vi "GUI_Frog_HPD_imagetester.vi"() -> ()   [LabVIEW 2013]
uses:
  Shared/GUI_Template/GUI_master/tcp_new_data_event.ctl
  Shared/GUI_Template/GUI_master/tcp new data cluster.ctl
  <vilib>/vision/Image Controls.llb/IMAQ Image.ctl
panel:
  out "www":T1(plugin-control)
  in  "retrievedFrogTrace::1":string caption="frogTrace::1"
  in  "frogTrace::1":string
  in  "triggermode::1":bool caption="Blank Button"
  out "test":T1(plugin-control) caption="Retrieved Frog Trace"
  in  "insert tag":bool=TRUE
  in  "stop":bool
  in  "GUIdevice 1":string="FrogHPD"
  out "tcp data event":T2
  out "error IO 2":errorcluster
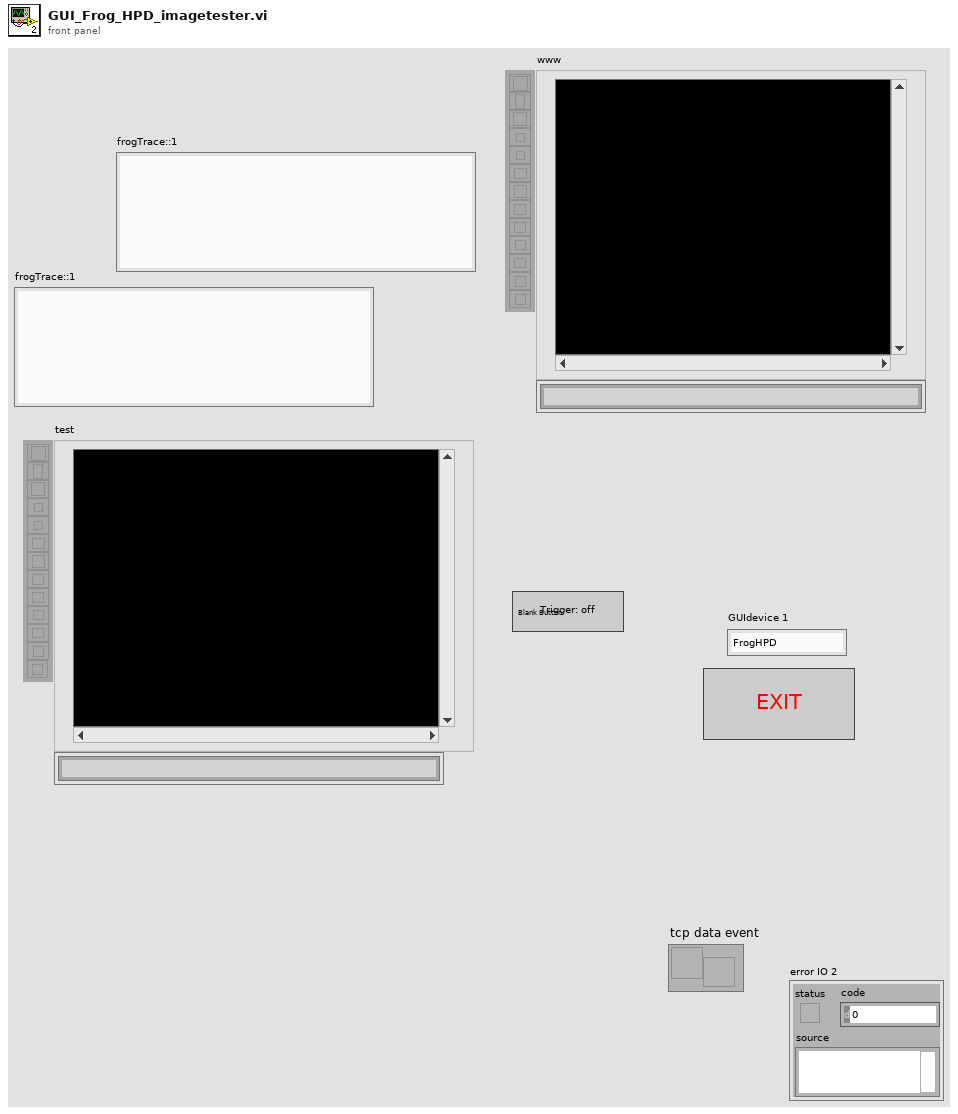
[diagram p1: front panel]
types:
  T1 = typedef "IMAQ Image.ctl" = refnum<image>
  T2 = typedef "tcp_new_data_event.ctl" = refnum<user-event>
  T3 = typedef "Image Type" = u32
  T4 = typedef "tcp new data cluster.ctl" = cluster{"EventEnum":enum16{"new data", "connection status update"}, "Device name":string}
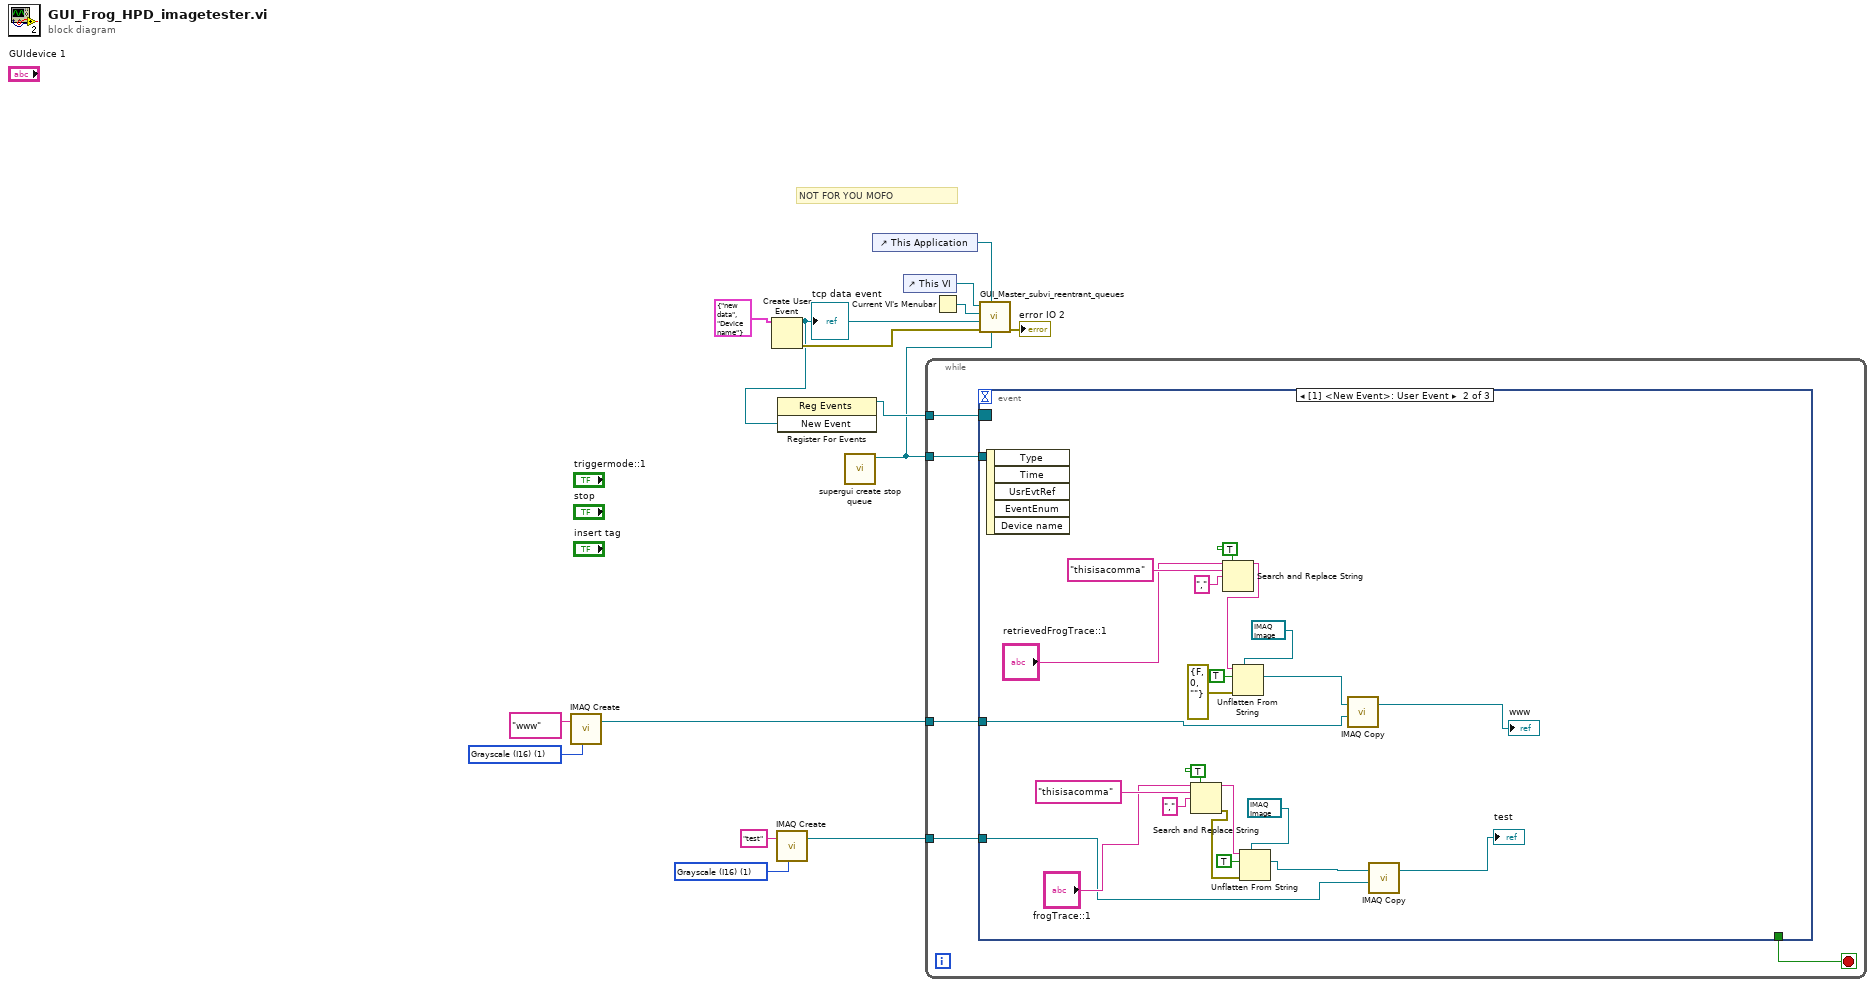
[diagram p0: block diagram]
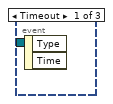
[diagram p2: hidden frame]
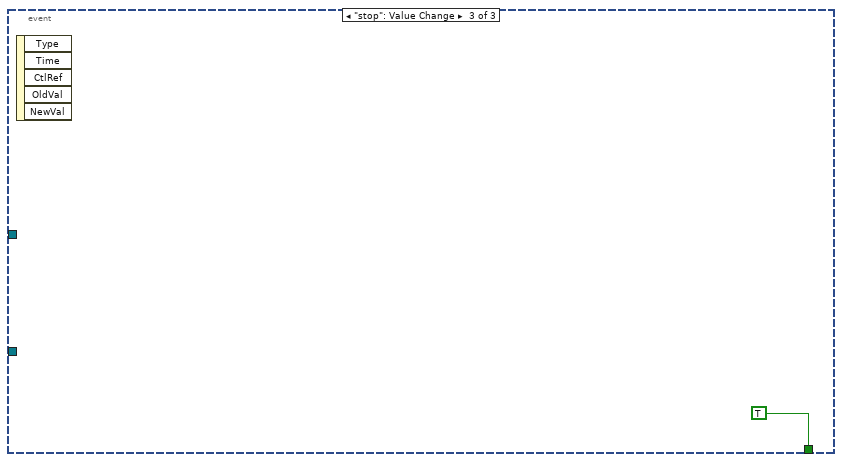
[diagram p3: hidden frame]
diagram:
  w3 = T3 1 items=["Grayscale (U8)", "Grayscale (I16)", "Grayscale (SGL)", "Complex (CSG)", "RGB (U32)", "HSL (U32)", "RGB (U64)", "Grayscale (U16)"] ("Image Type")
  w7 = T3 1 items=["Grayscale (U8)", "Grayscale (I16)", "Grayscale (SGL)", "Complex (CSG)", "RGB (U32)", "HSL (U32)", "RGB (U64)", "Grayscale (U16)"] ("Image Type")
  # "NOT FOR YOU MOFO"
  n1 = call "IMAQ Create"("Image Name"="www", "Image Type"=w7) -> ("New Image"=w5:T1)  [unwired: 3 in, 1 out]
  n2 = Create User Event(user event datatype=T4 {"EventEnum"=enum."new data", "Device name"="Device name"} ("New Event")) -> (user event=w9:refnum<user-event>, error out=w11:errorcluster)  [unwired: 1 in]
  "tcp data event" <- w9
  n3 = call "IMAQ Create"("Image Name"="test", "Image Type"=w3) -> ("New Image"=w2:T1)  [unwired: 3 in, 1 out]
  n4 = register-events(w9) -> (reference out=w8:refnum<event-registration>)  [unwired: 2 in, 1 out]
  n5 = call "supergui create stop queue.vi"() -> ("STOP Queue out"=w1:refnum<queue>)  [unwired: 11 in]
  n6 = control-ref of="This Application"() -> (w10:refnum<vi>)
  n7 = control-ref of="This VI"() -> (w14:refnum<vi>)
  n8 = while {
    tunnel: w8 -> [w19]
    tunnel: w5 -> [w18]
    tunnel: w2 -> [w17]
    tunnel: w1 -> [w16]
    stop <- w20 stop-if-true
    n9 = event shown="[1] <New Event>: User Event" {
      selector: w19 -> [_ _ _]
      dyn-events: _ -> [_ _ _]
      timeout: _ -> [_ _ _]
      tunnel: [_ _ TRUE] -> w20
      tunnel: w18 -> [_ w24 _]
      tunnel: w17 -> [_ w25 _]
      tunnel: w16 -> [_ _ _]
      event Timeout {
        n10 = event-data() -> ()  [unwired: 1 in, 2 out]
      }
      event User Event {
        n11 = event-data() -> ()  [unwired: 1 in, 5 out]
        n12 = Search and Replace String(replace all?=TRUE ("replace all? (F)"), input string="frogTrace::1", search string="thisisacomma", replace string="," ("replace string (\"\")")) -> (result string=w30:string, error out=w29:errorcluster)  [unwired: 4 in, 2 out]
        n13 = Search and Replace String(replace all?=TRUE ("replace all? (F)"), input string="retrievedFrogTrace::1", search string="thisisacomma", replace string="," ("replace string (\"\")")) -> (result string=w35:string)  [unwired: 4 in, 3 out]
        n14 = Unflatten From String(type=T1 refnum ("New Image"), binary string=w35, data includes array or string size? (T)=TRUE, error in (no error)=errorcluster {"status"=FALSE, "code"=0, "source"=""}) -> (value=w23:T1)  [unwired: 3 out]
        n15 = Unflatten From String(type=T1 refnum ("New Image"), binary string=w30, data includes array or string size? (T)=TRUE, error in (no error)=w29) -> (value=w28:T1)  [unwired: 3 out]
        n16 = call "IMAQ Copy"("Image Dst"=w24, "Image Src"=w23) -> ("Image Dst Out"=→"www":T1)  [unwired: 4 in, 1 out]
        n17 = call "IMAQ Copy"("Image Dst"=w25, "Image Src"=w28) -> ("Image Dst Out"=→"test":T1)  [unwired: 4 in, 1 out]
      }
      event "stop": Value Change {
        n18 = event-data() -> ()  [unwired: 1 in, 5 out]
      }
    }
  }
  n19 = Current VI's Menubar() -> (w13:refnum<k9>)
  n20 = call "GUI_Master_subvi_reentrant_queues.vi"("STOP Queue in"=w1, "This Application"=w10, "error in (no error)"=w11, "tcp data event"=w9, "Caller menu reference"=w13, "Caller VI ref"=w14) -> ("error out"=→"error IO 2":errorcluster)  [unwired: 5 in]
